vi "Setup.vi"(9 "Active Project":refnum<vi>, 10 "NI.LV.Dialog Instance":refnum<vi>) -> (2 "Found Target":string, 3 "Project Stuff out":refnum<class "Project Stuff.lvclass">)   [LabVIEW 2025, in "_Shared.lvlib" / "Project Stuff.lvclass"]
uses:
  Project Stuff.lvclass
  Refs.ctl
  VI.ctl
  Library.ctl
  Project Stuff.lvclass/Project Stuff.ctl
  <vilib>/Utility/EditLVProj/Edit LVProj.lvlib
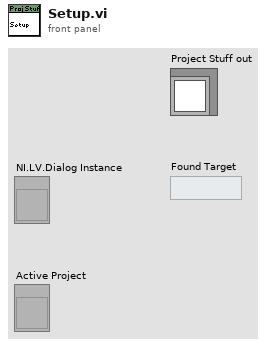
[diagram p1: front panel]
types:
  T1 = typedef "_Shared.lvlib/Project Stuff.lvclass/Library.ctl" = set{refnum<vi>}
  T2 = typedef "_Shared.lvlib/Project Stuff.lvclass/VI.ctl" = set{refnum<vi>}
  T3 = typedef "_Shared.lvlib/Project Stuff.lvclass/Refs.ctl" = cluster{"Target":refnum<vi>, "VI":T2, "Library":T1}
  T4 = typedef "Edit LVProj.lvlib/Library And VI References.ctl" = cluster{"Target Reference":refnum<vi>, "VI References":refnum<vi>[], "Library References":refnum<vi>[]}
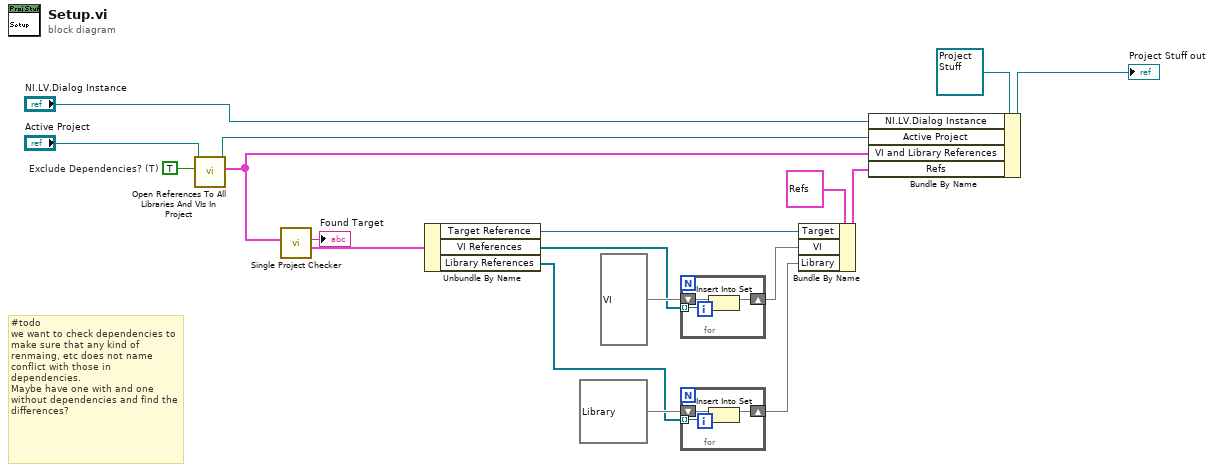
[diagram p0: block diagram]
diagram:
  w17 = TRUE  # Exclude Dependencies? (T)
  # "#todo\nwe want to check dependencies to make sure that any kind of renmaing, etc does not name conflict with those in dependencies.\nMaybe have one with and one without dependencies and find the differences?"
  n1 = call <vilib>:"Open References To All Libraries And VIs In Project.vi"("Exclude Dependencies? (T)"=w17, "Project in"="Active Project") -> ("VI and Library References"=w1:T4[], "Project out"=w18:refnum<vi>)  [unwired: 7 in, 1 out]
  n2 = call "Single Project Checker.vi"("VI and Library References"=w1) -> ("Ref"=w5:T4, "Found Target"=→"Found Target":string)  [unwired: 9 in]
  n3 = Unbundle By Name(w5) -> ("Target Reference"=w4:refnum<vi>, "VI References"=w8:refnum<vi>[], "Library References"=w6:refnum<vi>[])
  n4 = for {
    shift-right: [w20] -> w3
    shift-left: T2 {} ("VI") -> [w21]
    tunnel: w8 -> [w19] mode=indexing
    n5 = Insert Into Set(10:w19, 11:w21) -> (3:w20:T2)  [unwired: 1 out]
  }
  n6 = for {
    shift-right: [w23] -> w2
    shift-left: T1 {} ("Library") -> [w24]
    tunnel: w6 -> [w22] mode=indexing
    n7 = Insert Into Set(10:w22, 11:w24) -> (3:w23:T1)  [unwired: 1 out]
  }
  n8 = Bundle By Name(cluster=T3 {"Target"=refnum, "VI"={}, "Library"={}} ("Refs"), "Target"=w4, "VI"=w3, "Library"=w2) -> (w10:T3)
  n9 = Bundle By Name(cluster=refnum<class "Project Stuff.lvclass"> refnum ("Project Stuff out"), "NI.LV.Dialog Instance"="NI.LV.Dialog Instance", "Active Project"=w18, "VI and Library References"=w1, "Refs"=w10) -> (→"Project Stuff out":refnum<class "Project Stuff.lvclass">)
